vi "AttrMap-GetOrgKey.vi"(8 "error in (no error)":errorcluster, 10 "Key":string, 11 "AttrMap in":T1) -> (0 "error out":errorcluster, 2 "OrgKey String":string, 3 "AttrMap out":T1)   [LabVIEW 2019, in "lv-apt-json-file.lvlib"]
uses:
  lv-apt-json-file.lvlib
  Typedef/Def-AttrMap.ctl
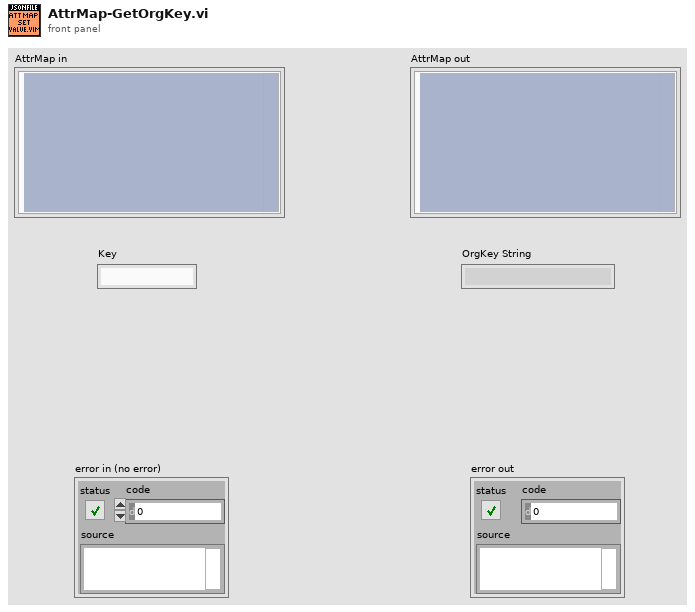
[diagram p1: front panel]
types:
  T1 = typedef "lv-apt-json-file.lvlib/Def-AttrMap.ctl" = cluster{"Map":variant}
  T2 = typedef "lv-apt-json-file.lvlib/Def-NameMap.ctl" = variant[]
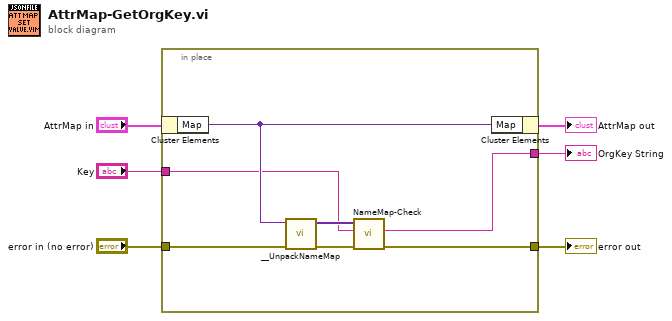
[diagram p0: block diagram]
diagram:
  n1 = in-place "In Place Element Structure" {
    in-place-border: "error in (no error)" -> [w10]
    in-place-border: [w9] -> w3
    in-place-border: "Key" -> [w8]
    in-place-border: [w7] -> w1
    n2 = in-place-cluster #1("AttrMap in") -> ("Map"=w11:variant)
    n3 = call "__UnpackNameMap.vi"("Map"=w11) -> ("NameMap"=w12:T2)  [unwired: 10 in]
    n4 = call "NameMap-Check.vi"("error in (no error)"=w10, "Name"=w8, "NameMap in"=w12) -> ("error out"=w9:errorcluster, "OriginName"=w7:string)  [unwired: 6 in, 1 out]
    n5 = in-place-cluster #1("Map"=w11) -> (→"AttrMap out":T1)
  }
  "error out" <- w3
  "OrgKey String" <- w1
